vi "Increment Time.vi"(8 "error in (no error)":errorcluster, 11 "Minutes in":i16) -> (0 "error out":errorcluster, 3 "Minutes out":i16)   [LabVIEW 2026]
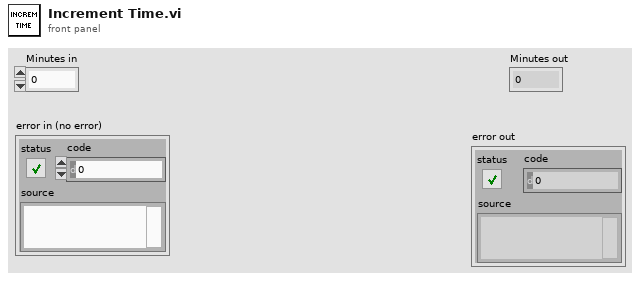
[diagram p1: front panel]
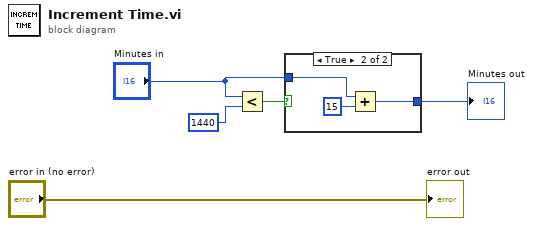
[diagram p0: block diagram]
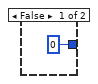
[diagram p2: hidden frame]
diagram:
  n1 = Less?(x="Minutes in", y=i16 1440) -> (x < y?=w4:bool)
  n2 = case shown="True" w4 {
    tunnel: [i16 0 w9] -> w1
    tunnel: "Minutes in" -> [_ w7]
    frame False {
    }
    frame True {
      n3 = Add(x=w7, y=i16 15) -> (x+y=w9:i16)
    }
  }
  "Minutes out" <- w1
  "error out" <- "error in (no error)"
